vi "simple_manual_trigger.vi"() -> ()   [LabVIEW 2011]
panel:
  out "trigger number":i32
  in  "cont. trigger":bool
  in  "milliseconds to wait":u32=100
  in  "number of triggers":i32
  in  "single trigger":bool
  in  "stop":bool
  in  "VISA resource name":refnum<visa-resource-name>="TRIG"
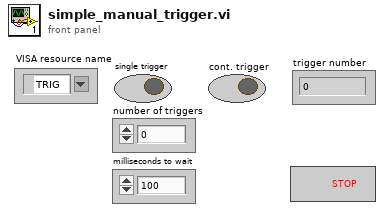
[diagram p1: front panel]
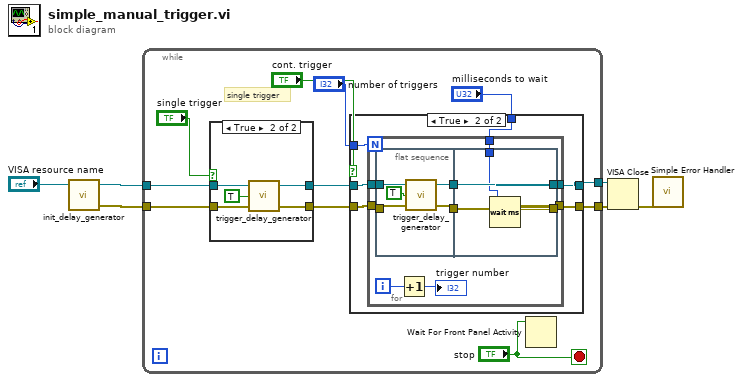
[diagram p0: block diagram]
diagram:
  n1 = call "init_delay_generator.vi"("VISA resource name"="VISA resource name") -> ("error out"=w4:errorcluster, "VISA resource name out"=w5:refnum<visa-resource-name>)  [unwired: 3 in]
  n2 = while {
    tunnel: w5 -> [w15]
    tunnel: w4 -> [w14]
    tunnel: [w11] -> w2
    tunnel: [w10] -> w1
    stop <- "stop" stop-if-true
    # "single trigger"
    n3 = case shown="True" "single trigger" {
      tunnel: w15 -> [w19 w24]
      tunnel: w14 -> [w18 w23]
      tunnel: [w19 w22] -> w13
      tunnel: [w18 w21] -> w12
      frame False {
      }
      frame True {
        n4 = call "trigger_delay_generator.vi"("error in (no error)"=w23, "Boolean"=TRUE, "VISA resource name"=w24) -> ("error out"=w21:errorcluster, "VISA resource name 2"=w22:refnum<visa-resource-name>)  [unwired: 1 in]
      }
    }
    n5 = case shown="True" "cont. trigger" {
      tunnel: w13 -> [w26 w32]
      tunnel: w12 -> [w25 w31]
      tunnel: [w26 w30] -> w11
      tunnel: [w25 w29] -> w10
      tunnel: "number of triggers" -> [_ w28]
      tunnel: "milliseconds to wait" -> [_ w27]
      frame False {
      }
      frame True {
        n6 = for {
          N: w28 -> [_]
          tunnel: w32 -> [w41]
          tunnel: w31 -> [w40]
          tunnel: [w39] -> w30
          tunnel: [w38] -> w29
          tunnel: w27 -> [w35]
          i -> [w34]
          n7 = flat-sequence {
            tunnel: w41 -> [w46]
            tunnel: w40 -> [w45]
            tunnel: [w44] -> w37
            tunnel: [w43] -> w36
            tunnel: [w48] -> w38
            tunnel: [w49] -> w39
            tunnel: w37 -> [w49]
            tunnel: w36 -> [w48]
            tunnel: w35 -> [w47]
            frame #0 {
              n8 = call "trigger_delay_generator.vi"("error in (no error)"=w45, "Boolean"=TRUE, "VISA resource name"=w46) -> ("error out"=w43:errorcluster, "VISA resource name 2"=w44:refnum<visa-resource-name>)  [unwired: 1 in]
            }
            frame #1 {
              n9 = Wait (ms)(milliseconds to wait=w47) -> ()  [unwired: 1 out]
            }
          }
          n10 = Increment(x=w34) -> (x+1=→"trigger number":i32)
        }
      }
    }
    n11 = Wait For Front Panel Activity(3:"stop") -> ()  [unwired: 2 in, 1 out]
  }
  n12 = VISA Close(VISA resource name=w2, error in (no error)=w1) -> (error out=w3:errorcluster)
  n13 = call <vilib>:"Simple Error Handler.vi"("error in (no error)"=w3) -> ()  [unwired: 4 in, 5 out]
